vi "Get Waveform Data Engine 2012 Workaround.vi"(8 "error in (no error)":errorcluster, 11 "Waveform Ref in":T1 format="%.0x") -> (0 "error out":errorcluster, 1 "Waveform":T2, 2 "Waveform Name":string, 3 "Waveform Ref out":T1 format="%.0x", 4 "Found":bool, 5 "GUID":string)   [LabVIEW 2015, in "Waveform Data Logger Engine.lvlib"]
uses:
  Waveform Data Logger Engine.lvlib
  <vilib>/NI Veristand/Custom Device API/Custom Device Waveform.ctl
  <vilib>/NI Veristand/Custom Device API/Custom Device Waveform DataType.ctl
  <vilib>/NI Veristand/Custom Device API/Custom Device Item Ref.ctl
  <vilib>/NI VeriStand/Custom Device API/Custom Device API.lvlib
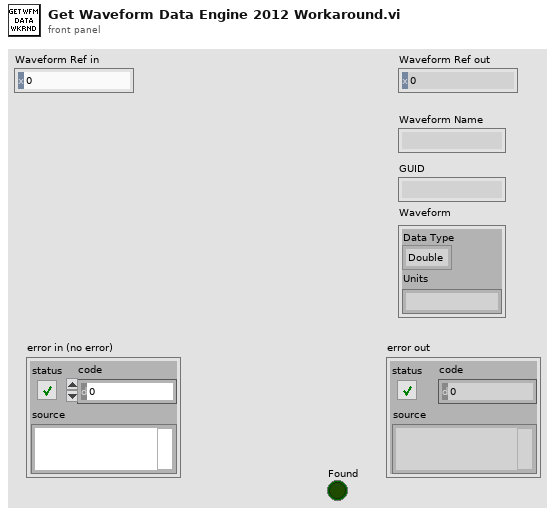
[diagram p1: front panel]
types:
  T1 = typedef "Custom Device API.lvlib/Custom Device Item Ref.ctl" = u64
  T2 = typedef "Custom Device API.lvlib/Custom Device Waveform.ctl" = cluster{"Data Type":T3, "Units":string}
  T3 = typedef "Custom Device API.lvlib/Custom Device Waveform DataType.ctl" = enum16{"Double", "Complex Double"}
  T4 = typedef "Binary Target System Storage.lvlib/Waveform Info.ctl" = cluster{"Units":string, "dataType":T5}
  T5 = typedef "WFMDataType.ctl" = i32
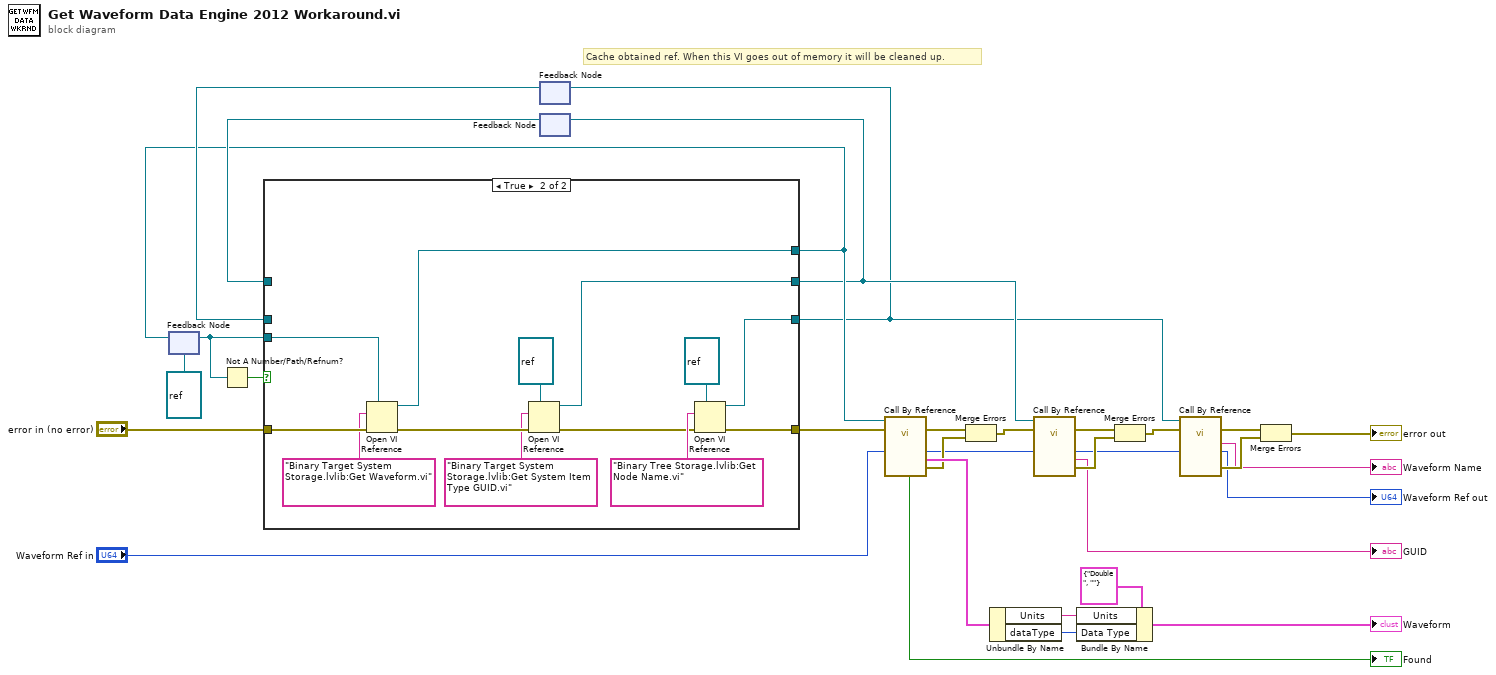
[diagram p0: block diagram]
diagram:
  # "Cache obtained ref. When this VI goes out of memory it will be cleaned up."
  n1 = feedback #1(refnum<vi> refnum ("type specifier VI Refnum (for type only)")) -> (w28:refnum<vi>)
  n2 = Not A Number/Path/Refnum?(number/path/refnum=w28) -> (NaN/Path/Refnum?=w31:bool)
  n3 = feedback #2() -> (w26:refnum<vi>)  [unwired: 1 in]
  n4 = feedback #3() -> (w27:refnum<vi>)  [unwired: 1 in]
  n5 = case shown="True" w31 {
    tunnel: "error in (no error)" -> [w34 w48]
    tunnel: w28 -> [w32 w47]
    tunnel: [w34 w39] -> w25
    tunnel: [w32 w38] -> w24
    tunnel: [w35 w37] -> w14
    tunnel: [w33 w36] -> w5
    tunnel: w27 -> [w35 _]
    tunnel: w26 -> [w33 _]
    frame False {
    }
    frame True {
      n6 = Open VI Reference(type specifier VI Refnum (for type only)=w47, vi path="Binary Target System Storage.lvlib:Get Waveform.vi", error in (no error)=w48) -> (vi reference=w38:refnum<vi>, error out=w45:errorcluster)  [unwired: 3 in]
      n7 = Open VI Reference(type specifier VI Refnum (for type only)=refnum<vi> refnum, vi path="Binary Target System Storage.lvlib:Get System Item Type GUID.vi", error in (no error)=w45) -> (vi reference=w37:refnum<vi>, error out=w40:errorcluster)  [unwired: 3 in]
      n8 = Open VI Reference(type specifier VI Refnum (for type only)=refnum<vi> refnum, vi path="Binary Tree Storage.lvlib:Get Node Name.vi", error in (no error)=w40) -> (vi reference=w36:refnum<vi>, error out=w39:errorcluster)  [unwired: 3 in]
    }
  }
  n9 = feedback-in #1(w24) -> ()
  n10 = feedback-in #2(w5) -> ()
  n11 = feedback-in #3(w14) -> ()
  n12 = call-by-ref "?"(reference=w24, error in=w25, "Base Node Ptr (0:Root)"="Waveform Ref in") -> (error out=w17:errorcluster, 0:"error out"=w16:errorcluster, "Waveform Info"=w22:T4, "System Item Node Ptr"=w13:u64, "Found"=→"Found":bool)  [unwired: 7 in, 1 out]
  n13 = Merge Errors(w17, w16) -> (w15:errorcluster)
  n14 = Unbundle By Name(w22) -> ("Units"=w20:string, "dataType"=w19:T5)
  n15 = call-by-ref "?"(reference=w14, error in=w15, "Base Node Index (0:Root)"=w13) -> (error out=w12:errorcluster, 0:"error out"=w11:errorcluster, "Type GUID"=→"GUID":string, "System Item Node Ptr"=w4:u64)  [unwired: 7 in, 2 out]
  n16 = Bundle By Name(cluster=T2 {"Data Type"=enum."Double", "Units"=""} ("Waveform"), "Units"=w20, "Data Type"=w19) -> (→"Waveform":T2)
  n17 = Merge Errors(w12, w11) -> (w6:errorcluster)
  n18 = call-by-ref "?"(reference=w5, error in=w6, "Node Ptr"=w4) -> (error out=w7:errorcluster, 0:"error out"=w8:errorcluster, "Node Ptr out"=→"Waveform Ref out":u64, "Node Name"=→"Waveform Name":string)  [unwired: 7 in, 2 out]
  n19 = Merge Errors(w7, w8) -> (→"error out":errorcluster)
